vi "RTB2Data.vi"(0 "inp":string) -> (1 "out1":dbl[](array[numeric]), 2 "out2":dbl[](array[numeric]), 3 "out3":dbl[](array[numeric]))   [LabVIEW 2019]
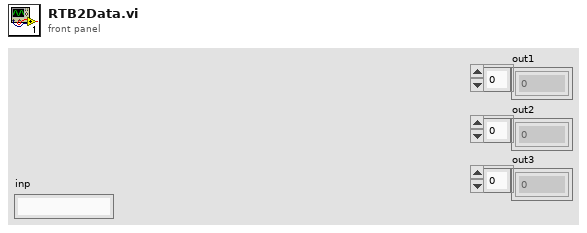
[diagram p1: front panel]
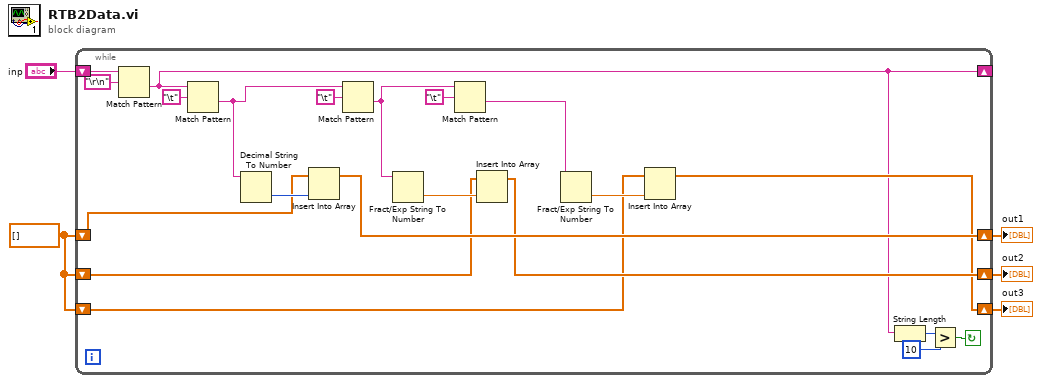
[diagram p0: block diagram]
diagram:
  w4 = dbl[] []
  n1 = while {
    shift-right: [w6] -> _
    shift-left: "inp" -> [w13]
    shift-right: [w14] -> w3
    shift-left: w4 -> [w15]
    shift-right: [w9] -> w2
    shift-left: w4 -> [w10]
    shift-right: [w7] -> w1
    shift-left: w4 -> [w8]
    stop <- w16 continue-if-true
    n2 = Match Pattern(string=w13, regular expression="\r\n") -> (after substring=w6:string)  [unwired: 1 in, 3 out]
    n3 = Match Pattern(string=w6, regular expression="\t") -> (after substring=w20:string)  [unwired: 1 in, 3 out]
    n4 = Decimal String To Number(string=w20) -> (number=w23:i32)  [unwired: 2 in, 1 out]
    n5 = Insert Into Array(array=w15, new element=w23) -> (w14:dbl[])  [unwired: 1 in]
    n6 = Match Pattern(string=w20, regular expression="\t") -> (after substring=w12:string)  [unwired: 1 in, 3 out]
    n7 = Fract/Exp String To Number(string=w12) -> (number=w11:dbl)  [unwired: 3 in, 1 out]
    n8 = Match Pattern(string=w12, regular expression="\t") -> (after substring=w18:string)  [unwired: 1 in, 3 out]
    n9 = Insert Into Array(array=w10, new element=w11) -> (w9:dbl[])  [unwired: 1 in]
    n10 = Fract/Exp String To Number(string=w18) -> (number=w17:dbl)  [unwired: 3 in, 1 out]
    n11 = Insert Into Array(array=w8, new element=w17) -> (w7:dbl[])  [unwired: 1 in]
    n12 = String Length(string=w6) -> (length=w25:i32)
    n13 = Greater?(x=w25, y=10) -> (0:w16:bool)
  }
  "out1" <- w3
  "out2" <- w2
  "out3" <- w1
